vi "CheckOutLogic.vi"(10 "Student ID":i32, 11 "Student List In":string[][](array[string])) -> (1 "Total Elapsed Time":i32, 2 "Total Seconds Out":string, 3 "Elapsed Seconds":i32)   [LabVIEW 2013]
doc: "Take current Hours, Minutes, Seconds, \nand Total Seconds, and add use to calculate \nthe difference between current time and the\n time at which the student checked in."
uses:
  Controls/SpreadsheetColumns.ctl
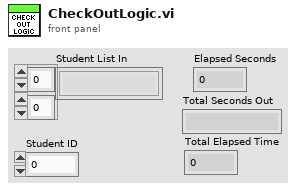
[diagram p1: front panel]
types:
  T1 = typedef "SpreadsheetColumns.ctl" = enum16{"Email", "CheckIn", "CheckOut", "Checkin Flag", "Hours", "Minutes", "Seconds", "Total Seconds", "Cat Points"}
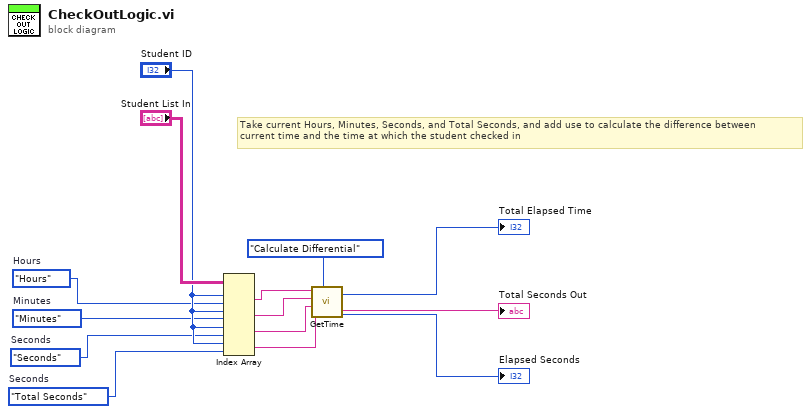
[diagram p0: block diagram]
diagram:
  w1 = SpreadsheetColumns."Total Seconds"  # Seconds
  w2 = SpreadsheetColumns."Seconds"  # Seconds
  w3 = SpreadsheetColumns."Minutes"  # Minutes
  w4 = SpreadsheetColumns."Hours"  # Hours
  # "Take current Hours, Minutes, Seconds, and Total Seconds, and add use to calculate the difference between\ncurrent time and the time at which the student checked in"
  n1 = Index Array(array="Student List In", index (row) #1="Student ID", index (col) #1=w4, index (row) #2="Student ID", index (col) #2=w3, index (row) #3="Student ID", index (col) #3=w2, index (row) #4="Student ID", index (col) #4=w1) -> (element #1=w10:string, element #2=w11:string, element #3=w12:string, element #4=w9:string)
  n2 = call "GetTime.vi"("State"=enum16{"Get Time", "Calculate Differential"}."Calculate Differential", "Total Seconds"=w9, "Stored Seconds"=w12, "Stored Minutes"=w11, "Stored Hours"=w10) -> ("Elapsed Seconds"=→"Elapsed Seconds":i32, "Total Seconds Out"=→"Total Seconds Out":string, "Total Elapsed Time"=→"Total Elapsed Time":i32)  [unwired: 1 in, 3 out]
